vi "Button to DIR.vi"(0 "Front":bool, 1 "Back":bool, 2 "Left":bool, 3 "Right":bool, 4 "Stop Button":bool) -> (5 "Direction 2":T1)   [LabVIEW 2015]
uses:
  Twin Shock/DIR GAME.ctl
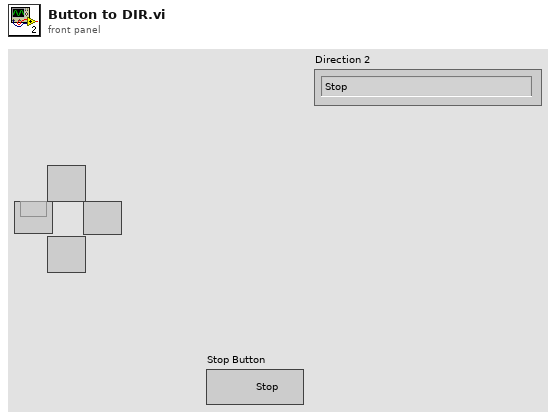
[diagram p1: front panel]
types:
  T1 = typedef "DIR GAME.ctl" = enum16{"Stop", "Front", "FR", "Right", "BR", "Back", "BL", "Left", "FL"}
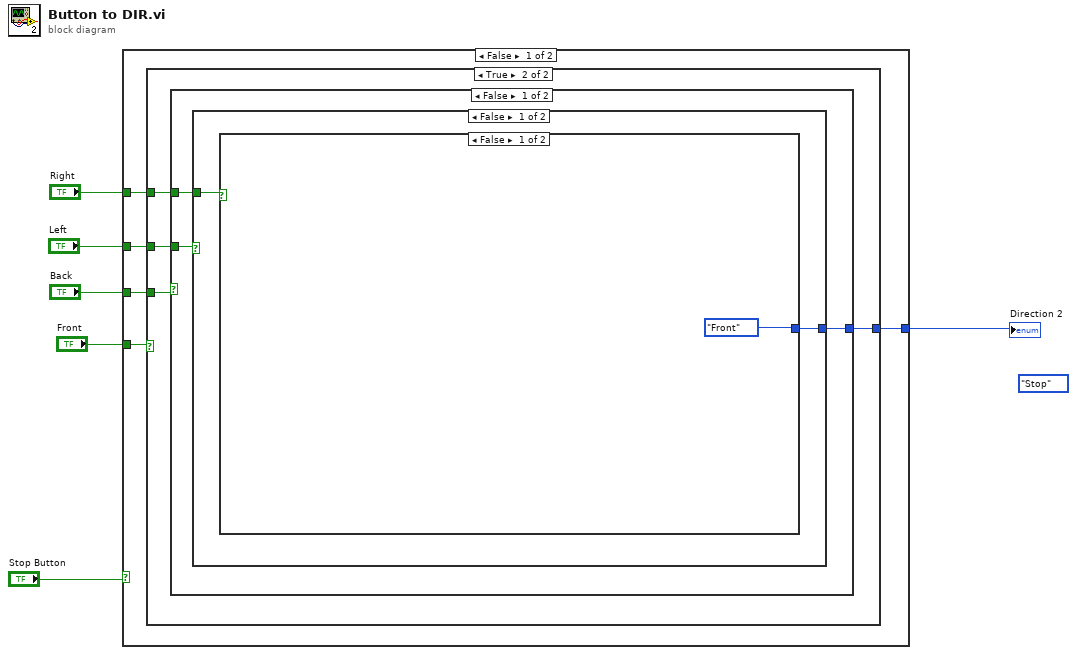
[diagram p0: block diagram]
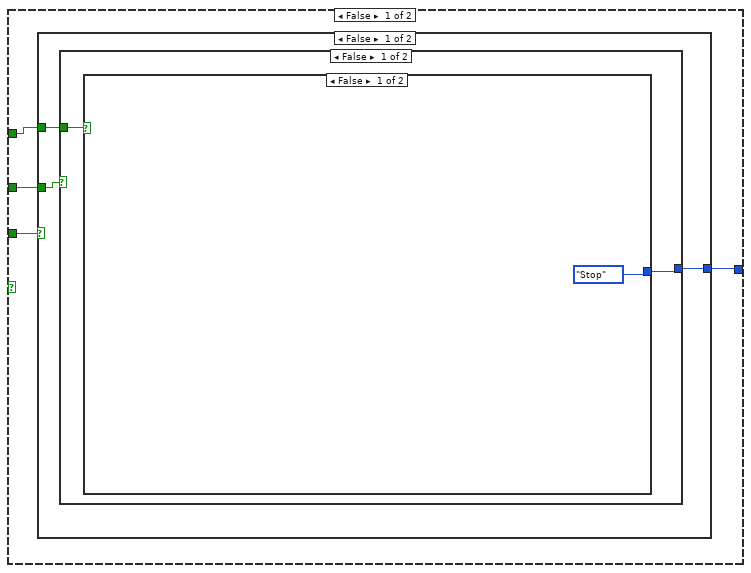
[diagram p2: hidden frame]
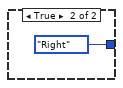
[diagram p3: hidden frame]
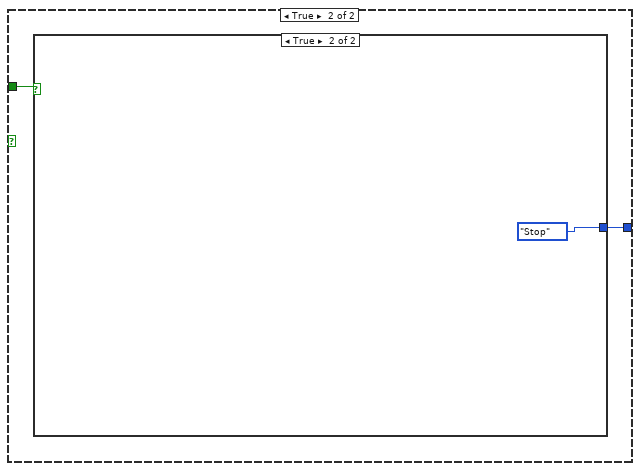
[diagram p4: hidden frame]
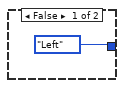
[diagram p5: hidden frame]
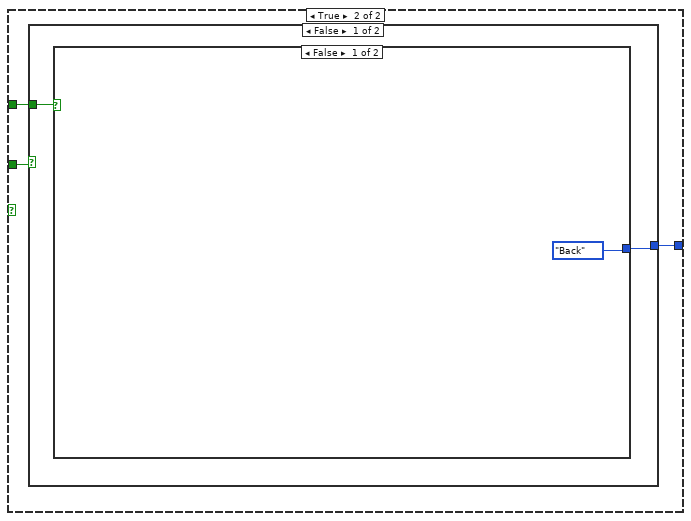
[diagram p6: hidden frame]
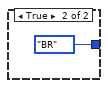
[diagram p7: hidden frame]
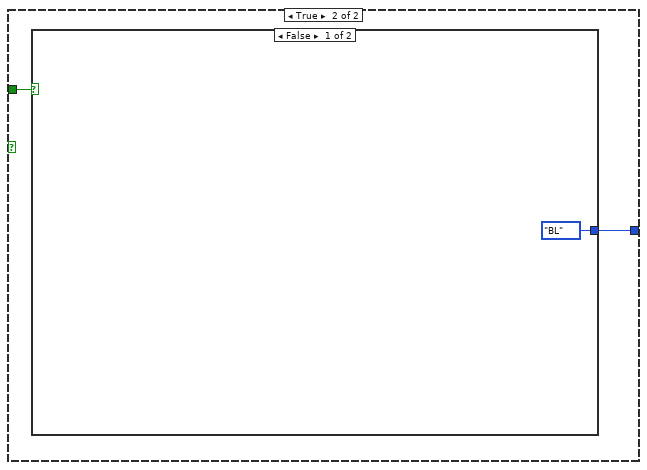
[diagram p8: hidden frame]
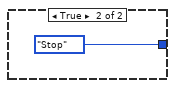
[diagram p9: hidden frame]
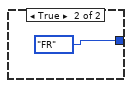
[diagram p10: hidden frame]
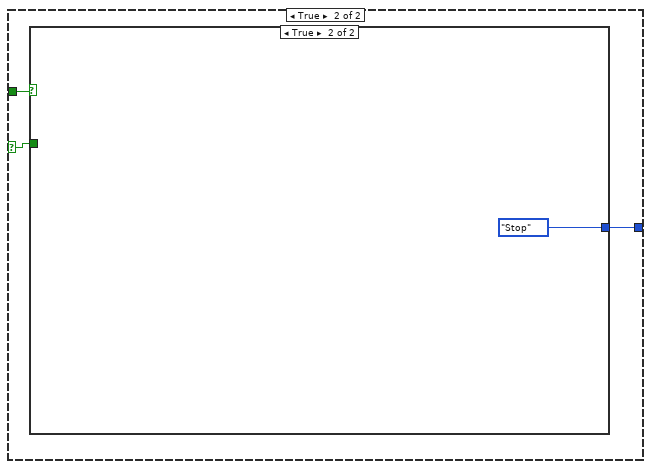
[diagram p11: hidden frame]
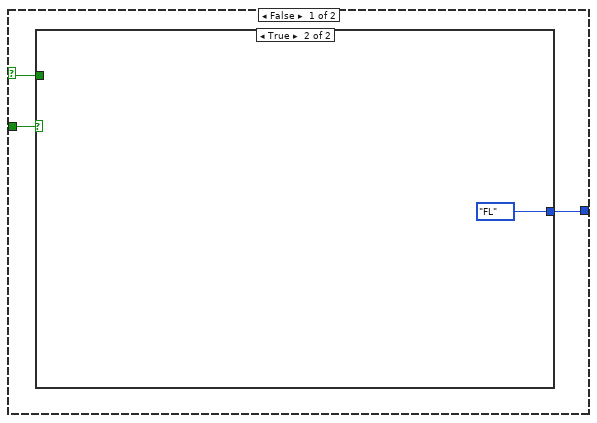
[diagram p12: hidden frame]
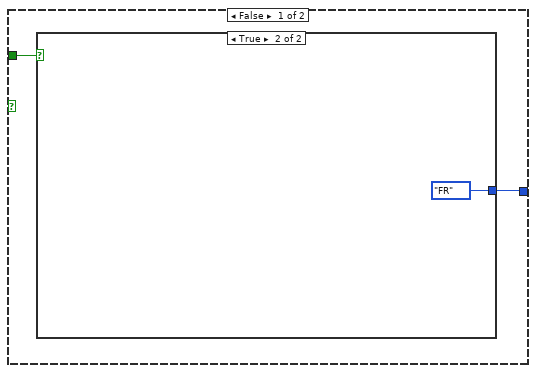
[diagram p13: hidden frame]
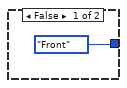
[diagram p14: hidden frame]
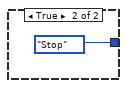
[diagram p15: hidden frame]
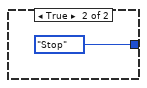
[diagram p16: hidden frame]
diagram:
  (unwired) DIR_GAME."Stop" ("Direction 3")
  n1 = case shown="False" "Stop Button" {
    tunnel: [w9 DIR_GAME."Stop" ("Direction 3")] -> w5
    tunnel: "Front" -> [w11 _]
    tunnel: "Back" -> [w10 _]
    tunnel: "Left" -> [w8 _]
    tunnel: "Right" -> [w7 _]
    frame False {
      n2 = case shown="True" w11 {
        tunnel: w10 -> [w15 w41]
        tunnel: [w12 w40] -> w9
        tunnel: w8 -> [w14 w39]
        tunnel: w7 -> [w13 w38]
        frame False {
          n3 = case shown="False" w15 {
            tunnel: w14 -> [w18 w29]
            tunnel: w13 -> [w17 w28]
            tunnel: [w16 w27] -> w12
            frame False {
              n4 = case shown="False" w18 {
                tunnel: w17 -> [w20 w24]
                tunnel: [w19 w23] -> w16
                frame False {
                  n5 = case shown="False" w20 {
                    tunnel: [DIR_GAME."Stop" ("Direction 3") DIR_GAME."Right" ("Direction 3")] -> w19
                    frame False {
                    }
                    frame True {
                    }
                  }
                }
                frame True {
                  n6 = case shown="True" w24 {
                    tunnel: [DIR_GAME."Left" ("Direction 3") DIR_GAME."Stop" ("Direction 3")] -> w23
                    frame False {
                    }
                    frame True {
                    }
                  }
                }
              }
            }
            frame True {
              n7 = case shown="False" w29 {
                tunnel: w28 -> [w31 w35]
                tunnel: [w30 w34] -> w27
                frame False {
                  n8 = case shown="False" w31 {
                    tunnel: [DIR_GAME."Back" ("Direction 3") DIR_GAME."BR" ("Direction 3")] -> w30
                    frame False {
                    }
                    frame True {
                    }
                  }
                }
                frame True {
                  n9 = case shown="False" w35 {
                    tunnel: [DIR_GAME."BL" ("Direction 3") DIR_GAME."Stop" ("Direction 3")] -> w34
                    frame False {
                    }
                    frame True {
                    }
                  }
                }
              }
            }
          }
        }
        frame True {
          n10 = case shown="False" w41 {
            tunnel: [w42 DIR_GAME."Stop" ("Direction 3")] -> w40
            tunnel: w39 -> [w44 _]
            tunnel: w38 -> [w43 _]
            frame False {
              n11 = case shown="False" w44 {
                selector: w44 -> [_ w49]
                tunnel: w43 -> [w46 w51]
                tunnel: [w45 w50] -> w42
                frame False {
                  n12 = case shown="False" w46 {
                    tunnel: [DIR_GAME."Front" ("Direction 3") DIR_GAME."FR" ("Direction 3")] -> w45
                    frame False {
                    }
                    frame True {
                    }
                  }
                }
                frame True {
                  n13 = case shown="True" w51 {
                    selector: w51 -> [w52 _]
                    tunnel: [w53 DIR_GAME."Stop" ("Direction 3")] -> w50
                    tunnel: w49 -> [w54 _]
                    frame False {
                      n14 = case shown="True" w54 {
                        tunnel: [w55 DIR_GAME."FL" ("Direction 3")] -> w53
                        tunnel: w52 -> [w56 _]
                        frame False {
                          n15 = case shown="True" w56 {
                            tunnel: [DIR_GAME."Front" ("Direction 3") DIR_GAME."FR" ("Direction 3")] -> w55
                            frame False {
                            }
                            frame True {
                            }
                          }
                        }
                        frame True {
                        }
                      }
                    }
                    frame True {
                    }
                  }
                }
              }
            }
            frame True {
            }
          }
        }
      }
    }
    frame True {
    }
  }
  "Direction 2" <- w5
